vi "Init.vi"(3 "Container State":T7, 4 "Previous State":variant, 5 "Previous Version":T6) -> (2 "Current State":T1)   [LabVIEW 2020, in "KTable.xctl"]
uses:
  KTable.xctl
  ColumnSpec.ctl
  ColumnType.ctl
  Table Properties.ctl
  Events.ctl
  Event Data.ctl
  Event Type.ctl
  <vilib>/_xctls/Container State.ctl
  <vilib>/_xctls/Version.ctl
  State V2.ctl
  State V3.ctl
  State V4.ctl
  State V5.ctl
  State V6.ctl
  State V7.ctl
  State V8.ctl
  <vilib>/_xctls/XControlSupport.lvlib
  State.ctl
panel:
  in  "Default Indicator State":T1
  in  "Default Control State":T1
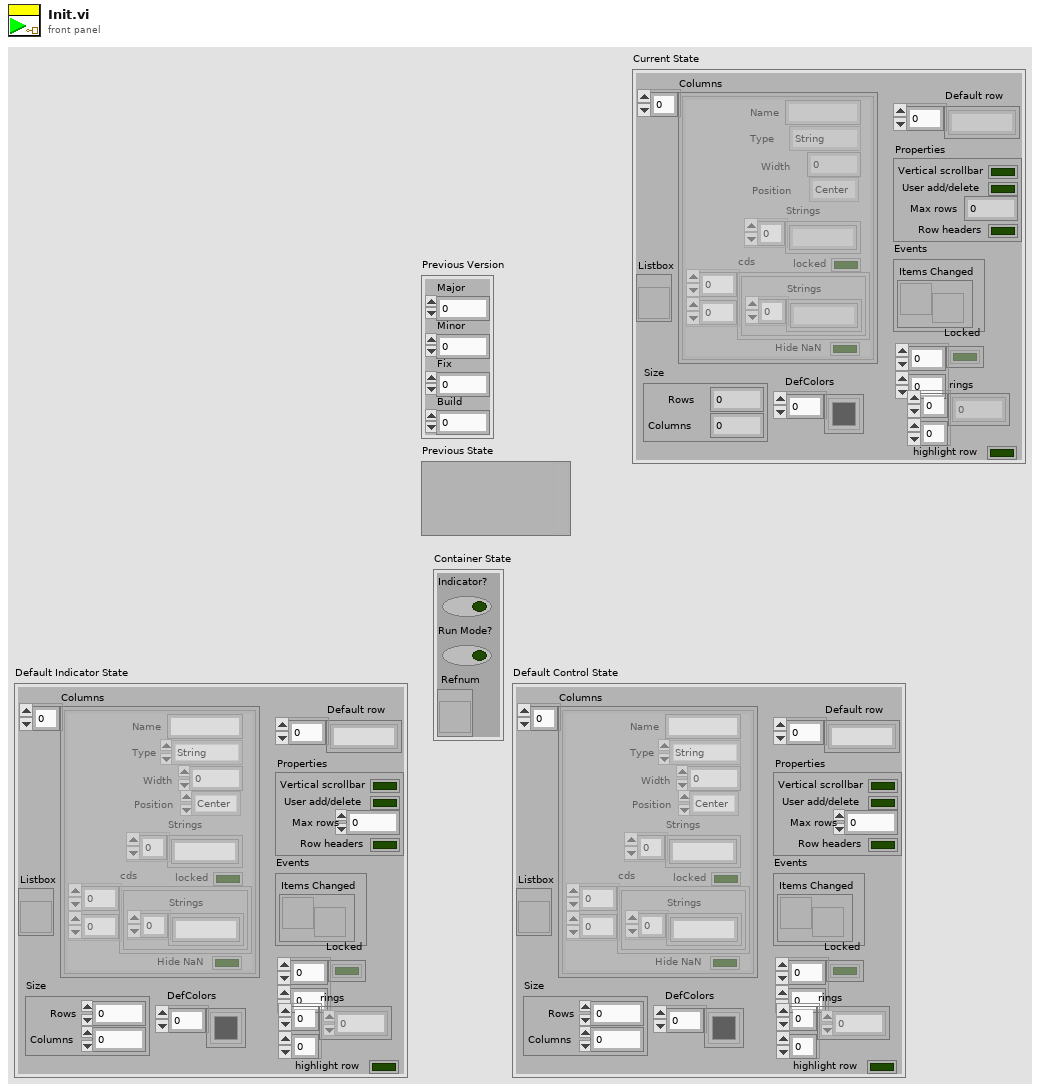
[diagram p1: front panel]
types:
  T1 = typedef "KTable.xctl/State.ctl" = cluster{"Columns":T2[], "Listbox":refnum<vi>, "Default row":string[], "Properties":T4, "Events":T5, "Locked":bool[][], "Size":cluster{"Rows":i32, "Columns":i32}, "rings":i32[][], "DefColors":u32[], "highlight row":bool}
  T2 = typedef "KTable.xctl/ColumnSpec.ctl" = cluster{"Name":string, "Type":T3, "Width":i32, "Strings":string[], "Position":enum16{"Left", "Center", "Right"}, "locked":bool, "cds":cluster{"Strings":string[]}[][], "Hide NaN":bool}
  T3 = typedef "KTable.xctl/ColumnType.ctl" = enum16{"String", "Enum", "Int", "Double", "Boolean", "Ring", "Formula", "Color"}
  T4 = typedef "KTable.xctl/Table Properties.ctl" = cluster{"Vertical scrollbar":bool, "User add/delete":bool, "Max rows":i32, "Row headers":bool}
  T5 = typedef "KTable.xctl/Events.ctl" = cluster{"Items Changed":refnum<user-event>}
  T6 = typedef "XControlSupport.lvlib/Version.ctl" = cluster{"Major":u16, "Minor":u16, "Fix":u16, "Build":u16}
  T7 = typedef "XControlSupport.lvlib/Container State.ctl" = cluster{"Indicator?":bool, "Run Mode?":bool, " Refnum":refnum<vi>}
  T8 = typedef "KTable.xctl/State V2.ctl" = cluster{"Columns":cluster{"Name":string, "Type":T3, "Width":i32, "Strings":string[], "Position":enum16{"Left", "Center", "Right"}}[], "Listbox":refnum<vi>, "Default row":string[], "Properties":T4, "Events":T5, "Locked":bool[][], "Size":cluster{"Rows":i32, "Columns":i32}}
  T9 = typedef "KTable.xctl/State V3.ctl" = cluster{"Columns":T2[], "Listbox":refnum<vi>, "Default row":string[], "Properties":cluster{"Vertical scrollbar":bool, "User add/delete":bool, "Max rows":i32}, "Events":T5, "Locked":bool[][], "Size":cluster{"Rows":i32, "Columns":i32}}
  T10 = typedef "KTable.xctl/State V4.ctl" = cluster{"Columns":cluster{"Name":string, "Type":T3, "Width":i32, "Strings":string[], "Position":enum16{"Left", "Center", "Right"}, "locked":bool}[], "Listbox":refnum<vi>, "Default row":string[], "Properties":T4, "Events":T5, "Locked":bool[][], "Size":cluster{"Rows":i32, "Columns":i32}}
  T11 = typedef "KTable.xctl/State V5.ctl" = cluster{"Columns":T2[], "Listbox":refnum<vi>, "Default row":string[], "Properties":T4, "Events":cluster{"Items Changed":refnum<user-event>}, "Locked":bool[][], "Size":cluster{"Rows":i32, "Columns":i32}, "rings":i32[][]}
  T12 = typedef "KTable.xctl/State V6.ctl" = cluster{"Columns":cluster{"Name":string, "Type":T3, "Width":i32, "Strings":string[], "Position":enum16{"Left", "Center", "Right"}, "locked":bool, "cds":cluster{"Strings":string[]}[][]}[], "Listbox":refnum<vi>, "Default row":string[], "Properties":T4, "Events":cluster{"Items Changed":refnum<user-event>}, "Locked":bool[][], "Size":cluster{"Rows":i32, "Columns":i32}, "rings":i32[][], "DefColors":u32[]}
  T13 = typedef "KTable.xctl/State V7.ctl" = cluster{"Columns":cluster{"Name":string, "Type":T3, "Width":i32, "Strings":string[], "Position":enum16{"Left", "Center", "Right"}, "locked":bool, "cds":cluster{"Strings":string[]}[][]}[], "Listbox":refnum<vi>, "Default row":string[], "Properties":cluster{"Vertical scrollbar":bool, "User add/delete":bool, "Max rows":i32, "Row headers":bool}, "Events":T5, "Locked":bool[][], "Size":cluster{"Rows":i32, "Columns":i32}, "rings":i32[][], "DefColors":u32[]}
  T14 = typedef "KTable.xctl/State V8.ctl" = cluster{"Columns":T2[], "Listbox":refnum<vi>, "Default row":string[], "Properties":T4, "Events":T5, "Locked":bool[][], "Size":cluster{"Rows":i32, "Columns":i32}, "rings":i32[][], "DefColors":u32[]}
  T15 = cluster{"Name":string, "Type":T3, "Width":i32, "Strings":string[], "Position":enum16{"Left", "Center", "Right"}}[]
  T16 = cluster{"Name":string, "Type":T3, "Width":i32, "Strings":string[], "Position":enum16{"Left", "Center", "Right"}, "locked":bool}[]
  T17 = cluster{"Name":string, "Type":T3, "Width":i32, "Strings":string[], "Position":enum16{"Left", "Center", "Right"}, "locked":bool, "cds":cluster{"Strings":string[]}[][]}[]
  T18 = cluster{"Vertical scrollbar":bool, "User add/delete":bool, "Max rows":i32, "Row headers":bool}
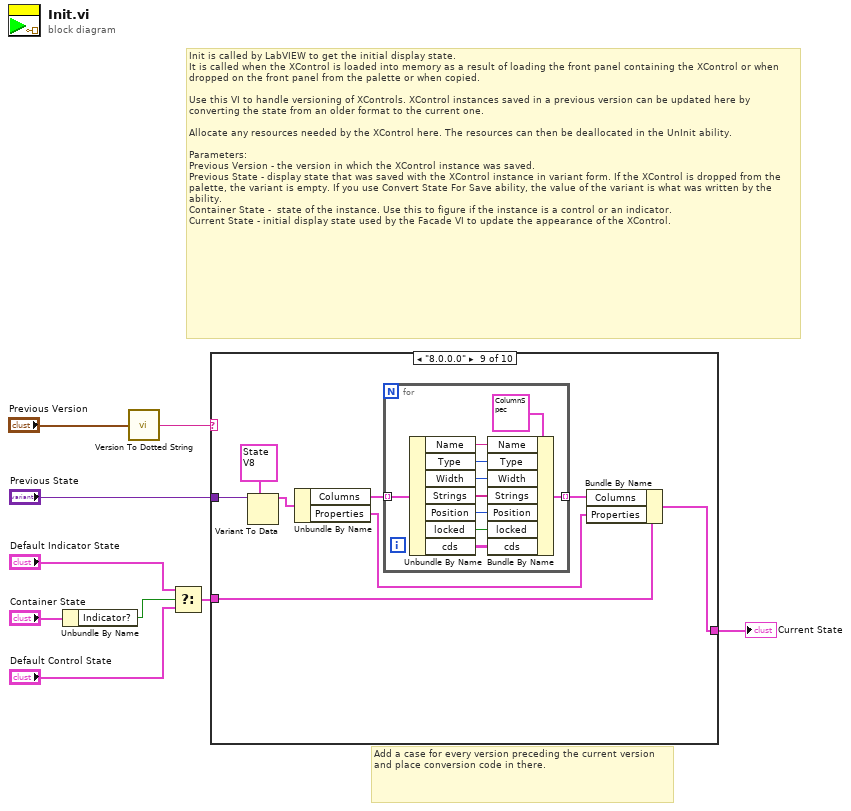
[diagram p0: block diagram]
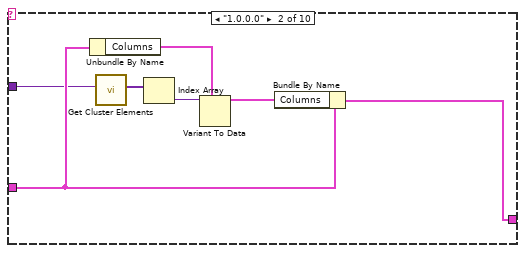
[diagram p3: hidden frame]
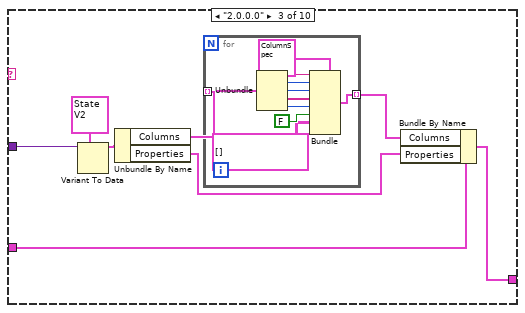
[diagram p4: hidden frame]
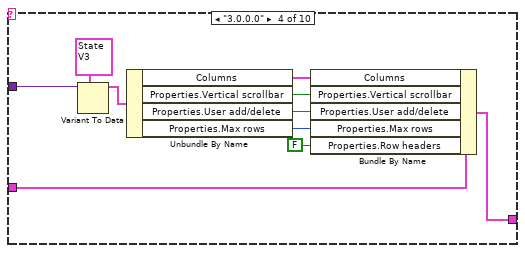
[diagram p5: hidden frame]
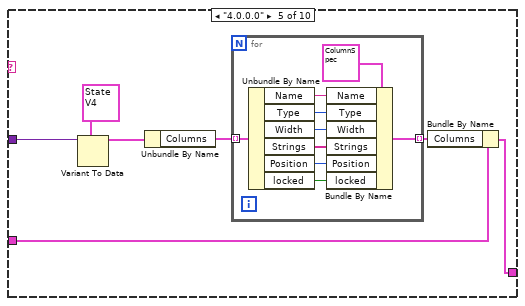
[diagram p6: hidden frame]
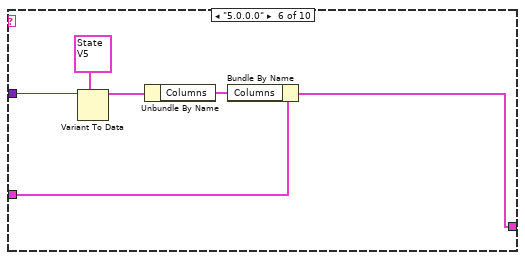
[diagram p7: hidden frame]
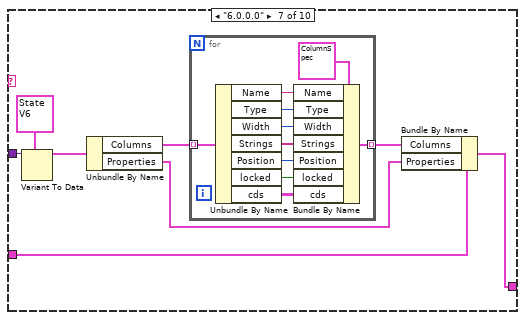
[diagram p8: hidden frame]
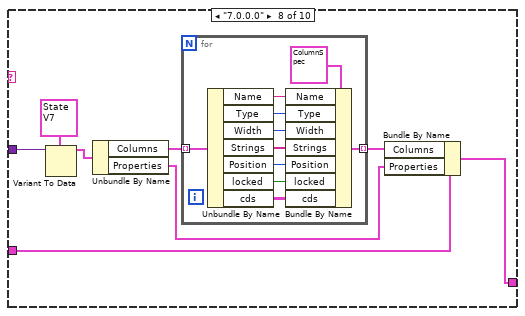
[diagram p9: hidden frame]
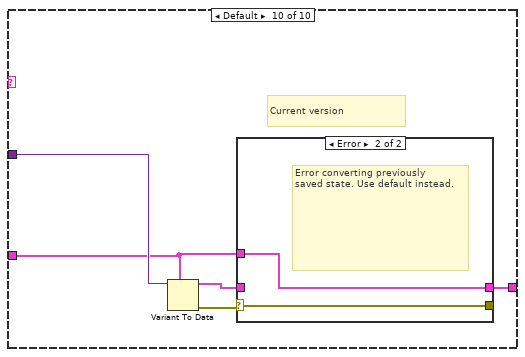
[diagram p10: hidden frame]
diagram:
  # "Add a case for every version preceding the current version and place conversion code in there."
  # "Init is called by LabVIEW to get the initial display state.\nIt is called when the XControl is loaded into memory as a result of loading the front panel containing the XControl or when dropped on the front panel from the palette or when copied.\n\nUse this VI to handle versioning of XControls. XControl instances saved in a previous version can be updated here by converting the state from an older format to the current one.\n\nAllocate any resources needed by the XControl here. The resources can then be deallocated in the UnInit ability.\n\nParameters:\nPrevious Version - the version in which the XControl instance was saved.\nPrevious State - display state that was saved with the XControl instance in variant form. If the XControl is dropped from the palette, the variant is empty. If you use Convert State For Save ability, the value of the variant is what was written by the ability. \nContainer State -  state of the instance. Use this to figure if the instance is a control or an indicator.\nCurrent State - initial display state used by the Facade VI to update the appearance of the XControl."
  n1 = Unbundle By Name("Container State") -> ("Indicator?"=w5:bool)
  n2 = call <vilib>:"Version To Dotted String.vi"("Version"="Previous Version") -> ("String Version"=w1:string)
  n3 = Select(t="Default Indicator State", s=w5, f="Default Control State") -> (s? t:f=w4:T1)
  n4 = case shown="\"8.0.0.0\"" w1 {
    tunnel: "Previous State" -> [_ w13 w23 w43 w50 w65 w73 w92 w110 w126]
    tunnel: [w10 w17 w25 w45 w52 w67 w75 w93 w111 w122] -> w2
    tunnel: w4 -> [w10 w14 w24 w44 w51 w66 w74 w88 w107 w123]
    frame "0.0.0.0" {
      # "Just created, use default state"
    }
    frame "1.0.0.0" {
      n5 = Unbundle By Name(w14) -> ("Columns"=w12:T2[])
      n6 = call "Get Cluster Elements.vi"("Cluster"=w13) -> ("Cluster Elements"=w16:variant[])  [unwired: 9 in, 1 out]
      n7 = Index Array(array=w16) -> (element=w15:variant)  [unwired: 1 in]
      n8 = Variant To Data(type=w12, Variant=w15) -> (data=w11:T2[])  [unwired: 1 in, 1 out]
      n9 = Bundle By Name(cluster=w14, "Columns"=w11) -> (w17:T1)
    }
    frame "2.0.0.0" {
      n10 = Variant To Data(type=T8 {"Columns"=[], "Listbox"=refnum, "Default row"=[], "Properties"={"Vertical scrollbar"=FALSE, "User add/delete"=FALSE, "Max rows"=0, "Row headers"=FALSE}, "Events"={"Items Changed"=refnum}, "Locked"=[], "Size"={"Rows"=0, "Columns"=0}} ("2.0.0.0"), Variant=w23) -> (data=w21:T8)  [unwired: 1 in, 1 out]
      n11 = Unbundle By Name(w21) -> ("Columns"=w19:T15, "Properties"=w20:T4)
      n12 = for {
        tunnel: w19 -> [w35] mode=indexing
        tunnel: [w28] -> w18 mode=indexing
        n13 = Unbundle(w35) -> ("Name"=w34:string, "Type"=w33:T3, "Width"=w32:i32, "Strings"=w31:string[], "Position"=w30:enum16{"Left", "Center", "Right"})
        n14 = Bundle(cluster=T2 {"Name"="", "Type"=enum."String", "Width"=0, "Strings"=[], "Position"=enum."Center", "locked"=FALSE, "cds"=[], "Hide NaN"=FALSE} ("ColSpec"), "Name"=w34, "Type"=w33, "Width"=w32, "Strings"=w31, "Position"=w30, "locked"=FALSE, "cds"=cluster{"Strings":string[]}[][] []) -> (w28:T2)  [unwired: 1 in]
      }
      n15 = Bundle By Name(cluster=w24, "Columns"=w18, "Properties"=w20) -> (w25:T1)
    }
    frame "3.0.0.0" {
      n16 = Variant To Data(type=T9 {"Columns"=[], "Listbox"=refnum, "Default row"=[], "Properties"={"Vertical scrollbar"=FALSE, "User add/delete"=FALSE, "Max rows"=0}, "Events"={"Items Changed"=refnum}, "Locked"=[], "Size"={"Rows"=0, "Columns"=0}} ("State"), Variant=w43) -> (data=w42:T9)  [unwired: 1 in, 1 out]
      n17 = Unbundle By Name(w42) -> ("Columns"=w41:T2[], "Properties.Vertical scrollbar"=w39:bool, "Properties.User add/delete"=w38:bool, "Properties.Max rows"=w37:i32)
      n18 = Bundle By Name(cluster=w44, "Columns"=w41, "Properties.Vertical scrollbar"=w39, "Properties.User add/delete"=w38, "Properties.Max rows"=w37, "Properties.Row headers"=FALSE) -> (w45:T1)
    }
    frame "4.0.0.0" {
      n19 = Variant To Data(type=T10 {"Columns"=[], "Listbox"=refnum, "Default row"=[], "Properties"={"Vertical scrollbar"=FALSE, "User add/delete"=FALSE, "Max rows"=0, "Row headers"=FALSE}, "Events"={"Items Changed"=refnum}, "Locked"=[], "Size"={"Rows"=0, "Columns"=0}} ("State"), Variant=w50) -> (data=w49:T10)  [unwired: 1 in, 1 out]
      n20 = Unbundle By Name(w49) -> ("Columns"=w47:T16)
      n21 = for {
        tunnel: w47 -> [w61] mode=indexing
        tunnel: [w59] -> w46 mode=indexing
        n22 = Unbundle By Name(w61) -> ("Name"=w57:string, "Type"=w58:T3, "Width"=w56:i32, "Strings"=w55:string[], "Position"=w54:enum16{"Left", "Center", "Right"}, "locked"=w53:bool)
        n23 = Bundle By Name(cluster=T2 {"Name"="", "Type"=enum."String", "Width"=0, "Strings"=[], "Position"=enum."Center", "locked"=FALSE, "cds"=[], "Hide NaN"=FALSE} ("ColSpec"), "Name"=w57, "Type"=w58, "Width"=w56, "Strings"=w55, "Position"=w54, "locked"=w53) -> (w59:T2)
      }
      n24 = Bundle By Name(cluster=w51, "Columns"=w46) -> (w52:T1)
    }
    frame "5.0.0.0" {
      n25 = Variant To Data(type=T11 {"Columns"=[], "Listbox"=refnum, "Default row"=[], "Properties"={"Vertical scrollbar"=FALSE, "User add/delete"=FALSE, "Max rows"=0, "Row headers"=FALSE}, "Events"={"Items Changed"=refnum}, "Locked"=[], "Size"={"Rows"=0, "Columns"=0}, "rings"=[]} ("State"), Variant=w65) -> (data=w64:T11)  [unwired: 1 in, 1 out]
      n26 = Unbundle By Name(w64) -> ("Columns"=w62:T2[])
      n27 = Bundle By Name(cluster=w66, "Columns"=w62) -> (w67:T1)
    }
    frame "6.0.0.0" {
      n28 = Variant To Data(type=T12 {"Columns"=[], "Listbox"=refnum, "Default row"=[], "Properties"={"Vertical scrollbar"=FALSE, "User add/delete"=FALSE, "Max rows"=0, "Row headers"=FALSE}, "Events"={"Items Changed"=refnum}, "Locked"=[], "Size"={"Rows"=0, "Columns"=0}, "rings"=[], "DefColors"=[]} ("State"), Variant=w73) -> (data=w72:T12)  [unwired: 1 in, 1 out]
      n29 = Unbundle By Name(w72) -> ("Columns"=w70:T17, "Properties"=w71:T4)
      n30 = for {
        tunnel: w70 -> [w85] mode=indexing
        tunnel: [w76] -> w69 mode=indexing
        n31 = Unbundle By Name(w85) -> ("Name"=w83:string, "Type"=w82:T3, "Width"=w81:i32, "Strings"=w80:string[], "Position"=w79:enum16{"Left", "Center", "Right"}, "locked"=w78:bool, "cds"=w77:cluster{"Strings":string[]}[][])
        n32 = Bundle By Name(cluster=T2 {"Name"="", "Type"=enum."String", "Width"=0, "Strings"=[], "Position"=enum."Center", "locked"=FALSE, "cds"=[], "Hide NaN"=FALSE} ("ColSpec"), "Name"=w83, "Type"=w82, "Width"=w81, "Strings"=w80, "Position"=w79, "locked"=w78, "cds"=w77) -> (w76:T2)
      }
      n33 = Bundle By Name(cluster=w74, "Columns"=w69, "Properties"=w71) -> (w75:T1)
    }
    frame "7.0.0.0" {
      n34 = Variant To Data(type=T13 {"Columns"=[], "Listbox"=refnum, "Default row"=[], "Properties"={"Vertical scrollbar"=FALSE, "User add/delete"=FALSE, "Max rows"=0, "Row headers"=FALSE}, "Events"={"Items Changed"=refnum}, "Locked"=[], "Size"={"Rows"=0, "Columns"=0}, "rings"=[], "DefColors"=[]} ("State"), Variant=w92) -> (data=w91:T13)  [unwired: 1 in, 1 out]
      n35 = Unbundle By Name(w91) -> ("Columns"=w89:T17, "Properties"=w86:T18)
      n36 = for {
        tunnel: w89 -> [w103] mode=indexing
        tunnel: [w94] -> w87 mode=indexing
        n37 = Unbundle By Name(w103) -> ("Name"=w101:string, "Type"=w100:T3, "Width"=w99:i32, "Strings"=w98:string[], "Position"=w97:enum16{"Left", "Center", "Right"}, "locked"=w96:bool, "cds"=w95:cluster{"Strings":string[]}[][])
        n38 = Bundle By Name(cluster=T2 {"Name"="", "Type"=enum."String", "Width"=0, "Strings"=[], "Position"=enum."Center", "locked"=FALSE, "cds"=[], "Hide NaN"=FALSE} ("ColSpec"), "Name"=w101, "Type"=w100, "Width"=w99, "Strings"=w98, "Position"=w97, "locked"=w96, "cds"=w95) -> (w94:T2)
      }
      n39 = Bundle By Name(cluster=w88, "Columns"=w87, "Properties"=w86) -> (w93:T1)
    }
    frame "8.0.0.0" {
      n40 = Variant To Data(type=T14 {"Columns"=[], "Listbox"=refnum, "Default row"=[], "Properties"={"Vertical scrollbar"=FALSE, "User add/delete"=FALSE, "Max rows"=0, "Row headers"=FALSE}, "Events"={"Items Changed"=refnum}, "Locked"=[], "Size"={"Rows"=0, "Columns"=0}, "rings"=[], "DefColors"=[]} ("State"), Variant=w110) -> (data=w109:T14)  [unwired: 1 in, 1 out]
      n41 = Unbundle By Name(w109) -> ("Columns"=w108:T2[], "Properties"=w105:T4)
      n42 = for {
        tunnel: w108 -> [w121] mode=indexing
        tunnel: [w112] -> w106 mode=indexing
        n43 = Unbundle By Name(w121) -> ("Name"=w119:string, "Type"=w118:T3, "Width"=w117:i32, "Strings"=w116:string[], "Position"=w115:enum16{"Left", "Center", "Right"}, "locked"=w114:bool, "cds"=w113:cluster{"Strings":string[]}[][])
        n44 = Bundle By Name(cluster=T2 {"Name"="", "Type"=enum."String", "Width"=0, "Strings"=[], "Position"=enum."Center", "locked"=FALSE, "cds"=[], "Hide NaN"=FALSE} ("ColSpec"), "Name"=w119, "Type"=w118, "Width"=w117, "Strings"=w116, "Position"=w115, "locked"=w114, "cds"=w113) -> (w112:T2)
      }
      n45 = Bundle By Name(cluster=w107, "Columns"=w106, "Properties"=w105) -> (w111:T1)
    }
    frame Default {
      # "Current version"
      n46 = Variant To Data(type=w123, Variant=w126) -> (data=w124:T1, error out=w125:errorcluster)  [unwired: 1 in]
      n47 = case shown="Error" w125 {
        selector: w125 -> [w128 w129]
        tunnel: w124 -> [w127 _]
        tunnel: [w127 w130] -> w122
        tunnel: w123 -> [_ w130]
        tunnel: [w128 w129] -> _
        frame No Error {
        }
        frame Error {
          # "Error converting previously \nsaved state. Use default instead."
        }
      }
    }
  }
  "Current State" <- w2
